vi "Analogue_overflow_checker.vi"(2 "I16 data":i16[][](array[numeric])) -> (0 "Over/Under string":string)   [LabVIEW 2010]
uses:
  Globals/Meas_global.vi
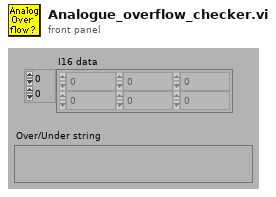
[diagram p1: front panel]
types:
  T1 = typedef "Board_Types.ctl" = enum16{"Simulate", "Local ADAM", "Server ADAM", "NI-DAQmx", "NI-DAQmxBase", "ADC488", "DT LV-link"}
  T2 = typedef "Ch_and_Spans.ctl" = cluster{"high limit (10V)":sgl, "low limit (-10V)":sgl, "Ch No":i16, "Var name":string, "Use Latest Calib":bool}
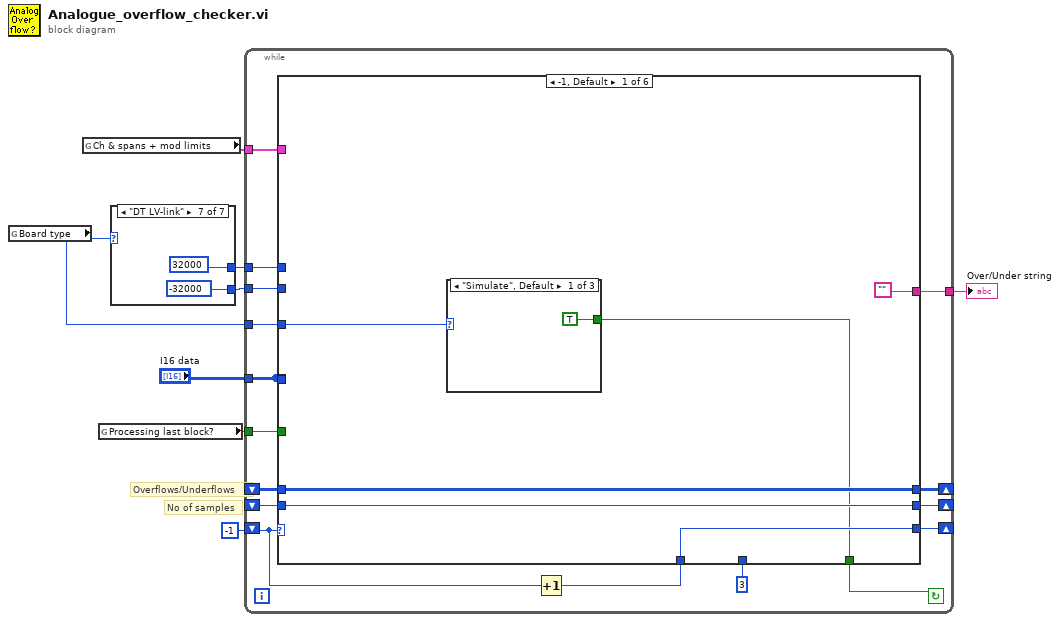
[diagram p0: block diagram]
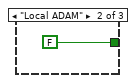
[diagram p2: hidden frame]
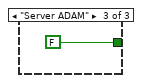
[diagram p3: hidden frame]
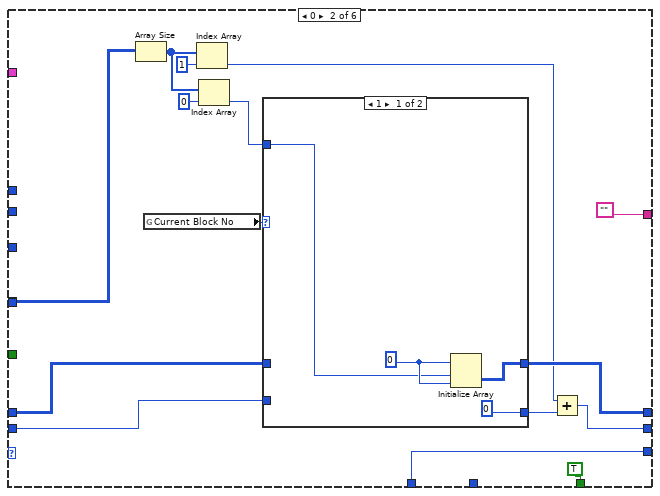
[diagram p4: hidden frame]
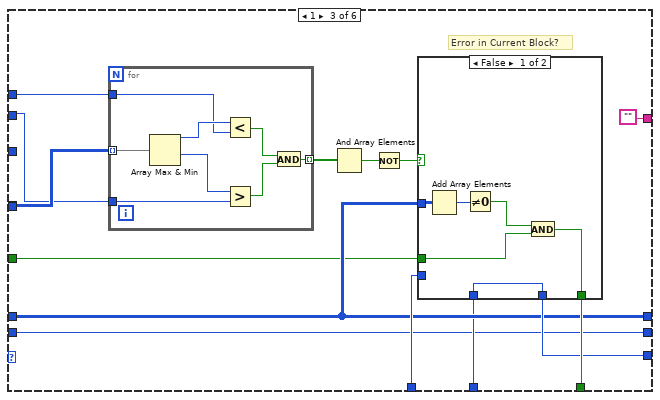
[diagram p6: hidden frame]
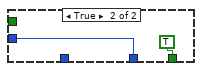
[diagram p7: hidden frame]
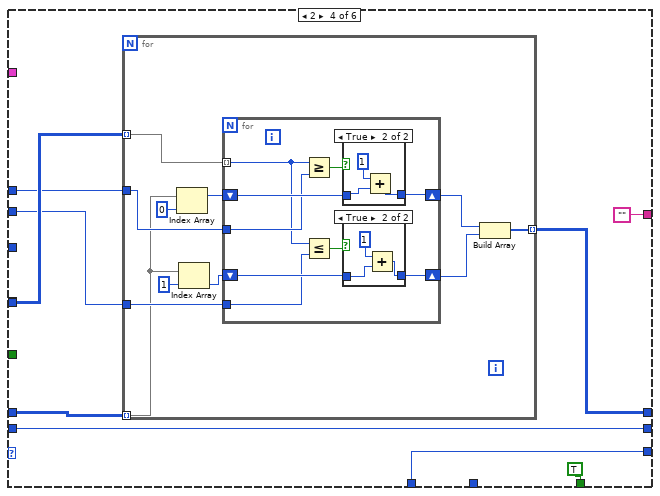
[diagram p8: hidden frame]
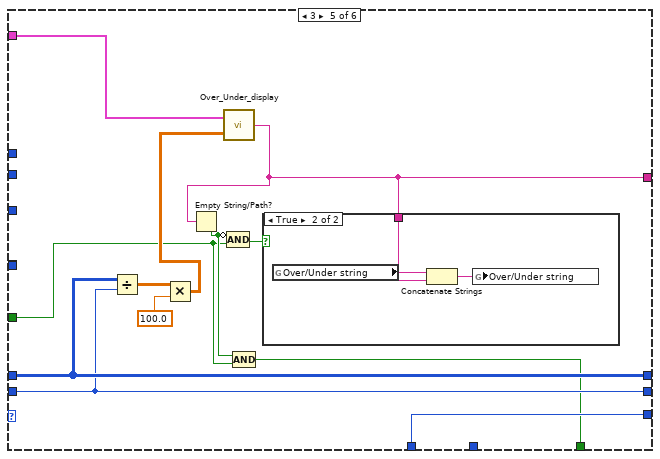
[diagram p11: hidden frame]
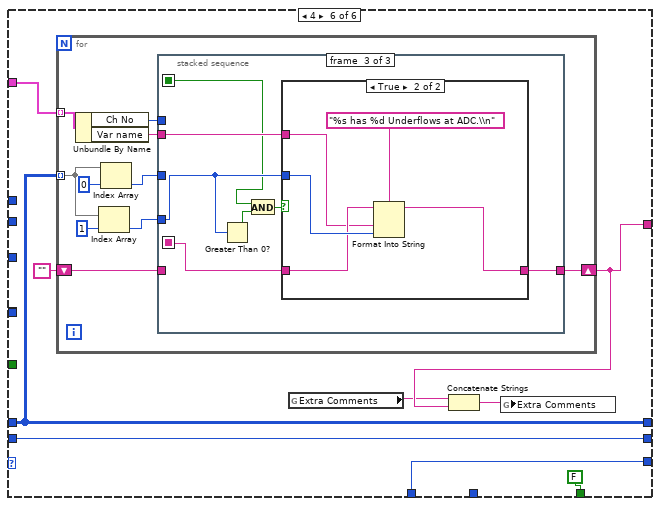
[diagram p13: hidden frame]
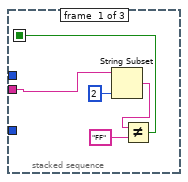
[diagram p14: hidden frame]
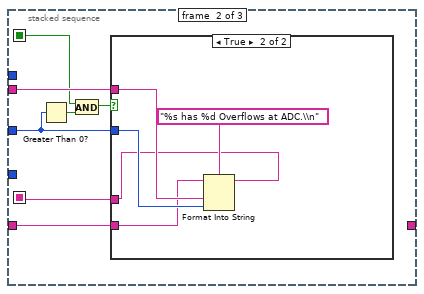
[diagram p15: hidden frame]
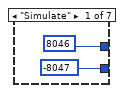
[diagram p18: hidden frame]
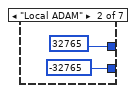
[diagram p19: hidden frame]
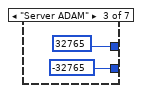
[diagram p20: hidden frame]
diagram:
  # "No of samples"
  # "Overflows/Underflows"
  n1 = global read "Meas_global.vi" "Board type"() -> (w2:T1)
  n2 = global read "Meas_global.vi" "Ch & spans + mod limits"() -> (w1:T2[])
  n3 = global read "Meas_global.vi" "Processing last block?"() -> (w4:bool)
  n4 = case shown="\"DT LV-link\"" w2 {
    tunnel: [i16 8046 i16 32765 i16 32765 i16 32000 i16 31500 i16 31500 i16 32000] -> w8
    tunnel: [i16 -8047 i16 -32765 i16 -32765 i16 -32000 i16 -31500 i16 -31500 i16 -32000] -> w7
    frame "Simulate" {
    }
    frame "Local ADAM" {
    }
    frame "Server ADAM" {
    }
    frame "NI-DAQmx" {
    }
    frame "NI-DAQmxBase" {
    }
    frame "ADC488" {
    }
    frame "DT LV-link" {
    }
  }
  n5 = while {
    tunnel: w2 -> [w23]
    tunnel: [w24] -> w3
    tunnel: w4 -> [w26]
    shift-left: _ -> [w30]
    shift-right: [w27] -> _
    shift-left: _ -> [w29]
    shift-right: [w28] -> _
    tunnel: "I16 data" -> [w31]
    shift-left: -1 -> [w34]
    shift-right: [w32] -> _
    tunnel: w7 -> [w36]
    tunnel: w8 -> [w37]
    tunnel: w1 -> [w38]
    stop <- w35 continue-if-true
    n6 = Increment(x=w34) -> (x+1=w33:i32)
    n7 = case shown="-1, Default" w34 {
      tunnel: w38 -> [_ _ _ _ w146 w154]
      tunnel: w37 -> [_ _ w81 w105 _ _]
      tunnel: w36 -> [_ _ w80 w106 _ _]
      tunnel: w31 -> [_ w54 w82 _ _ _]
      tunnel: [w39 TRUE w77 TRUE w136 FALSE] -> w35
      tunnel: w33 -> [w41 w57 w75 w103 w147 w159]
      tunnel: [w41 w57 w76 w103 w147 w159] -> w32
      tunnel: w31 -> [_ _ _ w107 _ _]
      tunnel: w30 -> [w42 w60 w71 w99 w144 w158]
      tunnel: w29 -> [w43 w58 w74 w100 w145 w155]
      tunnel: [w43 w61 w74 w104 w145 w155] -> w28
      tunnel: [w42 w51 w71 w99 w144 w158] -> w27
      tunnel: w26 -> [_ _ w69 _ w137 _]
      tunnel: 3 -> [_ _ w73 _ _ _]
      tunnel: ["" "" "" "" w139 w152] -> w24
      tunnel: w23 -> [w40 _ _ _ _ _]
      frame -1, Default {
        n8 = case shown="\"Simulate\", Default" w40 {
          tunnel: [TRUE FALSE FALSE] -> w39
          frame "Simulate", Default {
          }
          frame "Local ADAM" {
          }
          frame "Server ADAM" {
          }
        }
      }
      frame 0 {
        n9 = Array Size(array=w54) -> (size(s)=w49:i32[])
        n10 = global read "Meas_global.vi" "Current Block No"() -> (w62:i32)
        n11 = Index Array(array=w49, index=1 ("Index")) -> (element=w53:i32)
        n12 = Index Array(array=w49, index=0 ("Index")) -> (element=w48:i32)
        n13 = case shown="1" w62 {
          tunnel: [w66 w68] -> w61
          tunnel: w58 -> [_ w68]
          tunnel: w60 -> [_ w67]
          tunnel: [0 w67] -> w52
          tunnel: w48 -> [w63 _]
          frame 1 {
            w64 = 0
            n14 = Initialize Array(w64, w63, w64) -> (w66:i32[][])
          }
          frame 2, Default {
          }
        }
        n15 = Add(x=w53, y=w52) -> (x+y=w51:i32)
      }
      frame 1 {
        # "Error in Current Block?"
        n16 = for {
          tunnel: w82 -> [w98] mode=indexing
          tunnel: w81 -> [w96]
          tunnel: w80 -> [w94]
          tunnel: [w91] -> w79 mode=indexing
          n17 = Array Max & Min(array=w98) -> (max value=w97:i16, min value=w95:i16)  [unwired: 2 out]
          n18 = Less?(x=w97, y=w96) -> (x < y?=w92:bool)
          n19 = Greater?(x=w95, y=w94) -> (0:w93:bool)
          n20 = And(x=w92, y=w93) -> (x .and. y?=w91:bool)
        }
        n21 = And Array Elements(Boolean array=w79) -> (logical AND=w78:bool)
        n22 = Not(x=w78) -> (.not. x?=w70:bool)
        n23 = case shown="False" w70 {
          tunnel: [w84 TRUE] -> w77
          tunnel: [w83 w89] -> w76
          tunnel: w75 -> [_ w89]
          tunnel: w74 -> [w88 _]
          tunnel: w73 -> [w83 _]
          tunnel: w69 -> [w85 _]
          frame False {
            n24 = Add Array Elements(numeric array=w88) -> (sum=w87:i32)
            n25 = Not Equal To 0?(x=w87) -> (x != 0?=w86:bool)
            n26 = And(x=w86, y=w85) -> (x .and. y?=w84:bool)
          }
          frame True {
          }
        }
      }
      frame 2 {
        n27 = for {
          tunnel: w107 -> [w116] mode=indexing
          tunnel: w106 -> [w118]
          tunnel: w105 -> [w117]
          tunnel: [w114] -> w104 mode=indexing
          tunnel: w100 -> [w110] mode=indexing
          n28 = Index Array(array=w110, index=0 ("Index")) -> (element=w108:i32)
          n29 = Index Array(array=w110, index=1 ("Index")) -> (element=w109:i32)
          n30 = for {
            shift-right: [w122] -> w113
            shift-left: w109 -> [w123]
            shift-right: [w125] -> w115
            shift-left: w108 -> [w126]
            tunnel: w116 -> [w119] mode=indexing
            tunnel: w118 -> [w121]
            tunnel: w117 -> [w120]
            n31 = Greater Or Equal?(x=w119, y=w120) -> (x >= y?=w127:bool)
            n32 = Less Or Equal?(x=w119, y=w121) -> (x <= y?=w124:bool)
            n33 = case shown="True" w127 {
              tunnel: [w132 w134] -> w125
              tunnel: w126 -> [w132 w135]
              frame False {
              }
              frame True {
                n34 = Add(x=1, y=w135) -> (x+y=w134:i32)
              }
            }
            n35 = case shown="True" w124 {
              tunnel: w123 -> [w128 w130]
              tunnel: [w128 w129] -> w122
              frame False {
              }
              frame True {
                n36 = Add(x=1, y=w130) -> (x+y=w129:i32)
              }
            }
          }
          n37 = Build Array(w115, w113) -> (w114:i32[])
        }
      }
      frame 3 {
        n38 = Divide(x=w145, y=w144) -> (x/y=w143:dbl[][])
        n39 = Multiply(x=w143, y=100.0) -> (x*y=w141:dbl[][])
        n40 = call "Over_Under_display.vi"("Overflow array"=w141, "Ch & spans"=w146) -> ("Over/Under string"=w139:string)
        n41 = Empty String/Path?(string/path=w139) -> (empty?=w138:bool)
        n42 = Compound Arithmetic op=AND(invert w138, w137) -> (w140:bool)
        n43 = Compound Arithmetic op=AND(w138, w137) -> (w136:bool)
        n44 = case shown="True" w140 {
          tunnel: w139 -> [_ w148]
          frame False {
          }
          frame True {
            n45 = global read "Meas_global.vi" "Over/Under string"() -> (w150:string)
            n46 = Concatenate Strings(w150, w148) -> (w149:string)
            n47 = global write "Meas_global.vi" "Over/Under string"(w149) -> ()
          }
        }
      }
      frame 4 {
        n48 = for {
          tunnel: w154 -> [w169] mode=indexing
          tunnel: w155 -> [w168] mode=indexing
          shift-right: [w160] -> w152
          shift-left: "" -> [w161]
          n49 = Unbundle By Name(w169) -> ("Ch No"=w167:i16, "Var name"=w166:string)
          n50 = Index Array(array=w168, index=1) -> (element=w162:i32)
          n51 = Index Array(array=w168, index=0) -> (element=w163:i32)
          n52 = stacked-sequence {
            seq-local: [_ w179 _] -> [_ _ w194]
            seq-local: [w170 _ _] -> [_ w176 w188]
            tunnel: w162 -> [_ _ w192]
            tunnel: w163 -> [_ w178 _]
            tunnel: w166 -> [w171 w181 w191]
            tunnel: w167 -> [_ _ _]
            tunnel: w161 -> [_ w180 _]
            tunnel: [_ _ w193] -> w160
            frame #0 {
              n53 = String Subset(string=w171, length (rest)=2 ("length (rest)")) -> (substring=w173:string)  [unwired: 1 out]
              n54 = Not Equal?(x=w173, y="FF") -> (x != y?=w170:bool)
            }
            frame #1 {
              n55 = Greater Than 0?(x=w178) -> (x > 0?=w177:bool)
              n56 = And(x=w176, y=w177) -> (x .and. y?=w175:bool)
              n57 = case shown="True" w175 {
                tunnel: w178 -> [_ w185]
                tunnel: w181 -> [_ w186]
                tunnel: w180 -> [w182 w184]
                tunnel: [w182 w183] -> w179
                frame False {
                }
                frame True {
                  n58 = Format Into String(format string="%s has %d Overflows at ADC.\\n" ("Format String"), initial string=w184, w186, w185) -> (resulting string=w183:string)  [unwired: 1 in, 1 out]
                }
              }
            }
            frame #2 {
              n59 = Greater Than 0?(x=w192) -> (x > 0?=w190:bool)
              n60 = And(x=w188, y=w190) -> (x .and. y?=w189:bool)
              n61 = case shown="True" w189 {
                tunnel: w192 -> [_ w200]
                tunnel: w191 -> [_ w196]
                tunnel: w194 -> [w195 w199]
                tunnel: [w195 w198] -> w193
                frame False {
                }
                frame True {
                  n62 = Format Into String(format string="%s has %d Underflows at ADC.\\n" ("Format String"), initial string=w199, w196, w200) -> (resulting string=w198:string)  [unwired: 1 in, 1 out]
                }
              }
            }
          }
        }
        n63 = global read "Meas_global.vi" "Extra Comments"() -> (w151:string)
        n64 = Concatenate Strings(w151, w152) -> (w156:string)
        n65 = global write "Meas_global.vi" "Extra Comments"(w156) -> ()
      }
    }
  }
  "Over/Under string" <- w3
